vi "SMO.jsonRPC.SendSyncRequest.vi"(6 "timeout (50ms)":i32=50, 7 "Notification (F)":bool, 8 "error in (no error)":errorcluster, 9 "Parameters":variant, 10 "Method":string, 11 "SMO.jsonRPC in":refnum<class "SMO.jsonRPC.lvclass">) -> (0 "error out":errorcluster, 1 "id":i32, 2 "Response":refnum<class "Response.lvclass">, 3 "SMO.jsonRPC out":refnum<class "SMO.jsonRPC.lvclass">)   [LabVIEW 2013, in "SMO.jsonRPC.lvclass"]
uses:
  SMO.jsonRPC.lvclass
  <vilib>/JKI/JKI JSON RPC Specification/Response/Response.lvclass
  Typedefs/Request--Cluster.ctl
  <vilib>/JKI/JKI JSON RPC Specification/Request/Request.lvclass
  <vilib>/JKI/JKI JSON RPC Specification/Error/Error.lvclass
  <vilib>/addons/_JKI.lib/Serialization/JSON/JKI JSON Serialization.lvlib
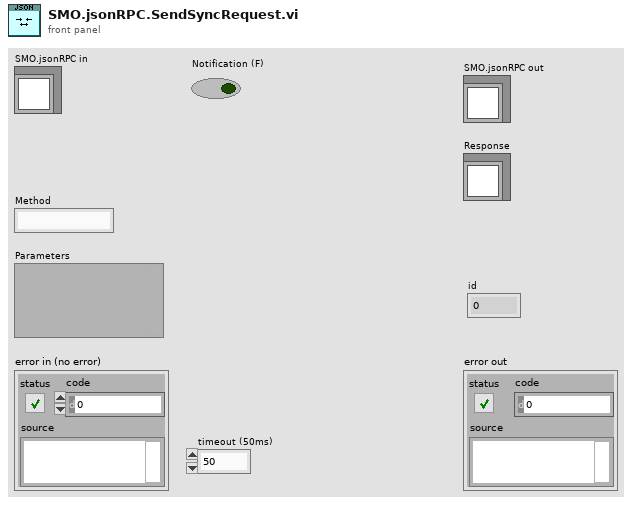
[diagram p1: front panel]
types:
  T1 = typedef "SMO.jsonRPC.lvclass/Request--Cluster.ctl" = cluster{"Request":refnum<class "Request.lvclass">, "reply queue":refnum<queue>, "Async?":bool}
  T2 = typedef "SMO.jsonRPC.lvclass/PrivateEvents--Cluster.ctl" = cluster{"Incoming Request":refnum<user-event>}
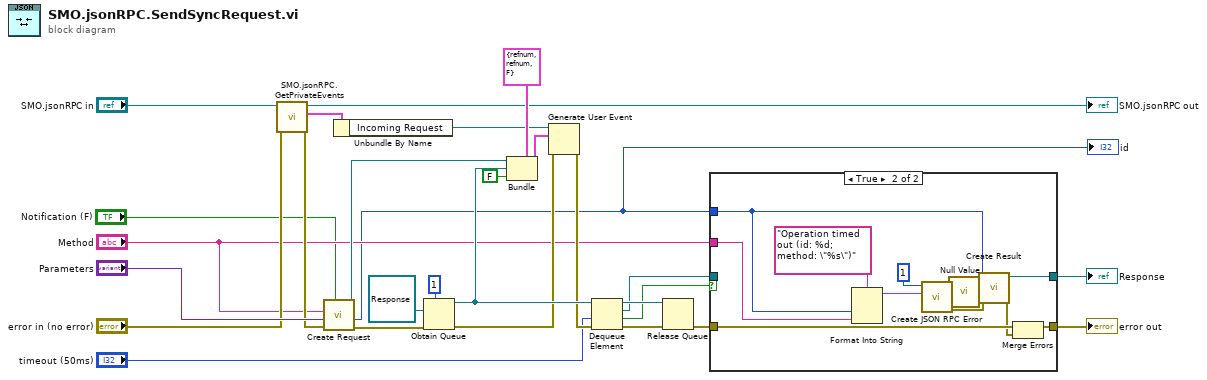
[diagram p0: block diagram]
diagram:
  n1 = call "SMO.jsonRPC.GetPrivateEvents.vi"("error in (no error)"="error in (no error)", "SMO.jsonRPC"="SMO.jsonRPC in") -> ("error out"=w26:errorcluster, "Private Events"=w11:T2, "SMO.jsonRPC out"=→"SMO.jsonRPC out":refnum<class "SMO.jsonRPC.lvclass">)  [unwired: 7 in]
  n2 = call <vilib>:"Create Request.vi"("Notification (F)"="Notification (F)", "error in (no error)"=w26, "Parameters"="Parameters", "Method"="Method") -> ("error out"=w24:errorcluster, "id"=w2:i32, "Request"=w23:refnum<class "Request.lvclass">)  [unwired: 4 in, 1 out]
  "id" <- w2
  n3 = Unbundle By Name(w11) -> ("Incoming Request"=w10:refnum<user-event>)
  n4 = Obtain Queue(max queue size (-1, unlimited)=1, element data type=refnum<class "Response.lvclass"> refnum ("Response"), error in (no error)=w24) -> (queue out=w20:refnum<queue>, error out=w14:errorcluster)  [unwired: 2 in, 1 out]
  n5 = Bundle(cluster=T1 {"Request"=refnum, "reply queue"=refnum, "Async?"=FALSE} ("event data"), "Request"=w23, "reply queue"=w20, "Async?"=FALSE) -> (w13:T1)
  n6 = Generate User Event(user event=w10, event data cluster=w13, error in=w14) -> (error out=w18:errorcluster)  [unwired: 1 in, 1 out]
  n7 = Dequeue Element(queue=w20, timeout in ms (-1)="timeout (50ms)", error in (no error)=w18) -> (queue out=w16:refnum<queue>, element=w7:refnum<class "Response.lvclass">, timed out?=w8:bool, error out=w17:errorcluster)
  n8 = Release Queue(queue=w16, error in (no error)=w17) -> (error out=w5:errorcluster)  [unwired: 1 in, 2 out]
  n9 = case shown="True" w8 {
    tunnel: w7 -> [w30 _]
    tunnel: [w30 w41] -> w6
    tunnel: w2 -> [_ w35]
    tunnel: w5 -> [w29 w38]
    tunnel: [w29 w39] -> w4
    tunnel: "Method" -> [_ w34]
    frame False {
    }
    frame True {
      n10 = Format Into String(format string="Operation timed out (id: %d; method: \"%s\")" ("Custom message"), w35, w34) -> (resulting string=w33:string)  [unwired: 2 in, 1 out]
      n11 = call <vilib>:"Create JSON RPC Error.vi"("Custom message"=w33, "JSON RPC Error"=1) -> ("error out"=w40:errorcluster, "Error out"=w42:refnum<class "Error.lvclass">)  [unwired: 7 in, 1 out]
      n12 = call <vilib>:"Null Value.vi"() -> ("Null"=w36:variant)
      n13 = call <vilib>:"Create Result.vi"("error in (no error)"=w40, "result"=w36, "Error"=w42, "id (-1: notification)"=w35) -> ("error out"=w37:errorcluster, "Response"=w41:refnum<class "Response.lvclass">)  [unwired: 5 in, 1 out]
      n14 = Merge Errors(w38, w37) -> (w39:errorcluster)
    }
  }
  "error out" <- w4
  "Response" <- w6
